vi "adapt_image.vi"(5 "captured image?":bool, 6 "crop (TRUE)":bool=TRUE, 8 "captImage_Y_Resolution":i32, 9 "captImage_X_Resolution":i32, 11 "orig_imageIn":T1) -> (0 "u8_ar_mask":u8[][](array[numeric]), 1 "adapted image px array":u8[][](array[numeric]), 3 "adapted image":T1)   [LabVIEW 2011]
doc: "Crops an image (original or captured) to cubic format (x-resolution = y-resolution) and applies a circular mask. Cropping and masking can be corrected using the crop-correction and mask-correction inputs.\n\nIf the input image is original (captured image set to FALSE) the image size will be adapted to match the size of the captured image and the image is flipped along the horizontal axis to account for the mirror image."
uses:
  <vilib>/vision/Image Controls.llb/IMAQ Image.ctl
  global_vars.vi
  <vilib>/vision/NI_Vision_Development_Module.lvlib
panel:
  in  "captured image? 2":bool
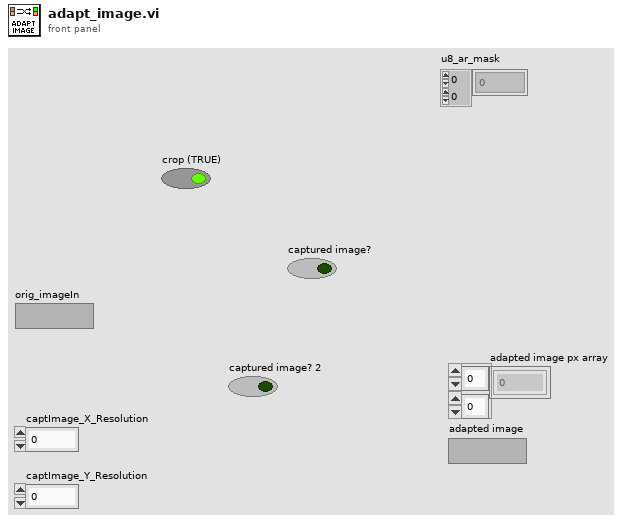
[diagram p1: front panel]
types:
  T1 = typedef "IMAQ Image.ctl" = refnum<image>
  T2 = cluster{"radius correction":i16, "u8_x_center_cor":i16, "u8_y_center_cor":i16}
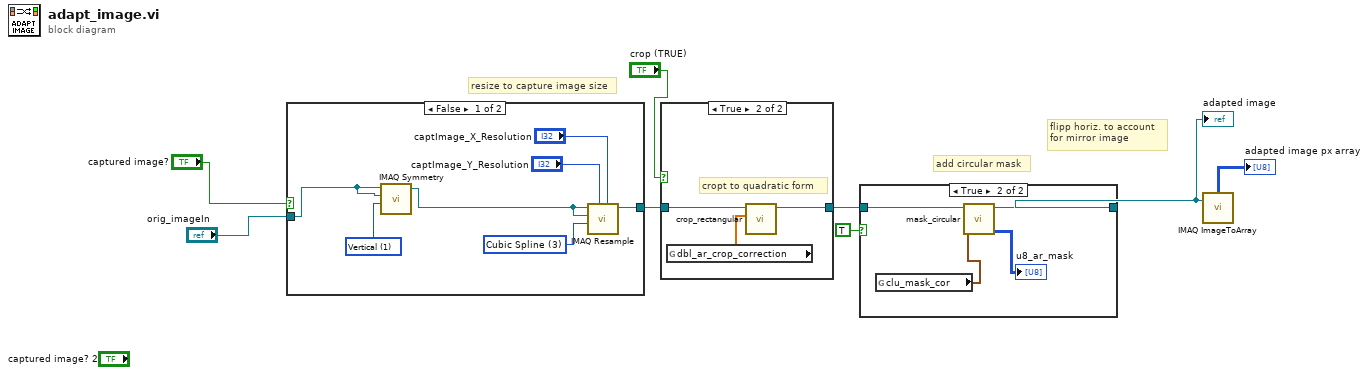
[diagram p0: block diagram]
diagram:
  # "flipp horiz. to account\nfor mirror image"
  # "resize to capture image size"
  # "add circular mask"
  n1 = case shown="False" "captured image?" {
    tunnel: [w13 w16] -> w8
    tunnel: "orig_imageIn" -> [w9 w16]
    frame False {
      w10 = u32 1 items=["Horizontal", "Vertical", "Central", "1st Diagonal", "2nd Diagonal"] ("Type of Symmetry")
      w12 = u32 3 items=["Zero Order", "Bi-Linear", "Quadratic", "Cubic Spline"] ("Interpolation Type")
      n2 = call "IMAQ Symmetry"("Type of Symmetry"=w10, "Image Dst"=w9, "Image Src"=w9) -> ("Image Dst Out"=w11:T1)  [unwired: 2 in, 1 out]
      n3 = call "IMAQ Resample"("X Resolution"="captImage_X_Resolution", "Y Resolution"="captImage_Y_Resolution", "Interpolation Type"=w12, "Image Dst"=w11, "Image Src"=w11) -> ("Image Dst Out"=w13:T1)  [unwired: 5 in, 1 out]
    }
    frame True {
    }
  }
  n4 = case shown="True" "crop (TRUE)" {
    tunnel: w8 -> [w17 w20]
    tunnel: [w17 w19] -> w6
    frame False {
    }
    frame True {
      # "cropt to quadratic form"
      n5 = global read "global_vars.vi" "dbl_ar_crop_correction"() -> (w18:dbl[])
      n6 = call "crop_rectangular.vi"("dbl_ar_crop_correction"=w18, "image_in"=w20) -> ("cropped image out"=w19:T1)  [unwired: 8 in, 1 out]
    }
  }
  n7 = case shown="True" TRUE {
    tunnel: w6 -> [w21 w25]
    tunnel: [w21 w24] -> w5
    frame False {
    }
    frame True {
      n8 = global read "global_vars.vi" "clu_mask_cor"() -> (w23:T2)
      n9 = call "mask_circular.vi"("clu_mask_cor"=w23, "image in"=w25) -> ("u8_ar_mask"=→"u8_ar_mask":u8[][], "masekd image out"=w24:T1)  [unwired: 8 in]
    }
  }
  "adapted image" <- w5
  n10 = call "IMAQ ImageToArray"("Image"=w5) -> ("Image Pixels (U8)"=→"adapted image px array":u8[][])  [unwired: 3 in, 4 out]
